vi "Force Create Task.vi"(8 "error in (no error)":errorcluster, 11 "Task Name":string) -> (0 "error out":errorcluster, 3 "Task out":refnum<k21>)   [LabVIEW 2021, in "Load Frame.lvlib"]
uses:
  Load Frame.lvlib
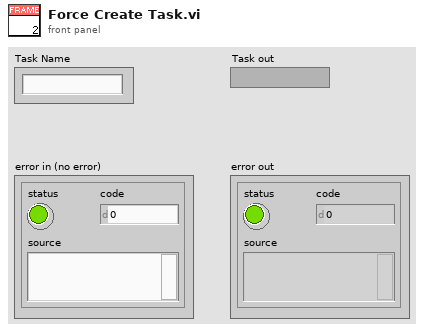
[diagram p1: front panel]
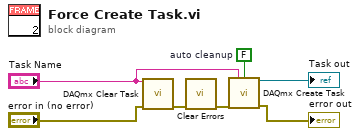
[diagram p0: block diagram]
diagram:
  w4 = FALSE  # auto cleanup
  n1 = call <vilib>:"DAQmx Clear Task.vi"("task in"="Task Name", "error in"="error in (no error)") -> ("error out"=w2:errorcluster)  [unwired: 13 in]
  n2 = call <vilib>:"Clear Errors.vi"("error in (no error)"=w2) -> ("error out"=w1:errorcluster)  [unwired: 5 in, 1 out]
  n3 = call <vilib>:"DAQmx Create Task.vi"("new task name"="Task Name", "auto cleanup"=w4, "error in"=w1) -> ("task out"=→"Task out":refnum<k21>, "error out"=→"error out":errorcluster)  [unwired: 11 in]
